vi "User ManualV1.vi"() -> ()   [LabVIEW 2020, in "Exaprom PDF.lvlib"]
uses:
  <userlib>/labview-PDF-writer-master/Exaprom PDF.lvlib
  <userlib>/labview-PDF-writer-master/Controls/Initialization Controls/Captions.ctl
  <userlib>/labview-PDF-writer-master/Controls/Initialization Controls/Image or Table Caption.ctl
  <userlib>/labview-PDF-writer-master/Controls/Font Controls/Font complete cluster.ctl
  <userlib>/labview-PDF-writer-master/Controls/Font Controls/Font size.ctl
  <userlib>/labview-PDF-writer-master/Controls/Font Controls/Font color.ctl
  <userlib>/labview-PDF-writer-master/Controls/Font Controls/Type and encoding.ctl
  <userlib>/labview-PDF-writer-master/Controls/Text Controls/Unicode/Type and run direction.ctl
  <userlib>/labview-PDF-writer-master/Controls/Initialization Controls/At the opening.ctl
  <userlib>/labview-PDF-writer-master/Controls/Initialization Controls/Defaut Paragraphe and Line Spacing.ctl
  <userlib>/labview-PDF-writer-master/Controls/Text Controls/Texte alignement.ctl
  <userlib>/labview-PDF-writer-master/Controls/Text Controls/Line spacing.ctl
  <userlib>/labview-PDF-writer-master/Controls/Initialization Controls/Unit.ctl
  <userlib>/labview-PDF-writer-master/Controls/Page Controls/Page setup.ctl
  <userlib>/labview-PDF-writer-master/Controls/Page Controls/Page size.ctl
  <userlib>/labview-PDF-writer-master/Controls/Page Controls/Page Orientation.ctl
  <userlib>/labview-PDF-writer-master/Controls/Page Controls/Page Layout Custom.ctl
  <userlib>/labview-PDF-writer-master/Controls/Page Controls/Page margins.ctl
  <userlib>/labview-PDF-writer-master/Controls/Image Controls/Image border.ctl
  <userlib>/labview-PDF-writer-master/Controls/Image Controls/Image alignment and position.ctl
  <userlib>/labview-PDF-writer-master/Controls/Image Controls/Image aligment.ctl
  <vilib>/measure/NI_MABase.lvlib
panel:
  out "波形图表":waveform(dbl)(graph)
  in  "Captions":T1={"Figure"={"Caption"="Figure", "Separator"=" QWE ", "Position"=enum."Below"}, "Table"={"Caption"="Table", "Separator"="  ", "Position"=enum."Above"}, "Font"={"Name"="", "Size"=-1.0, "Color"=0, "Style"={"Bold"=FALSE, "Italic"=FALSE, "Underline"=FALSE, "Strikeout"=FALSE}, "Type"={"Type&direction"=enum."Select", "Embedded"=FALSE, "Encoding"=""}}} caption="标题"
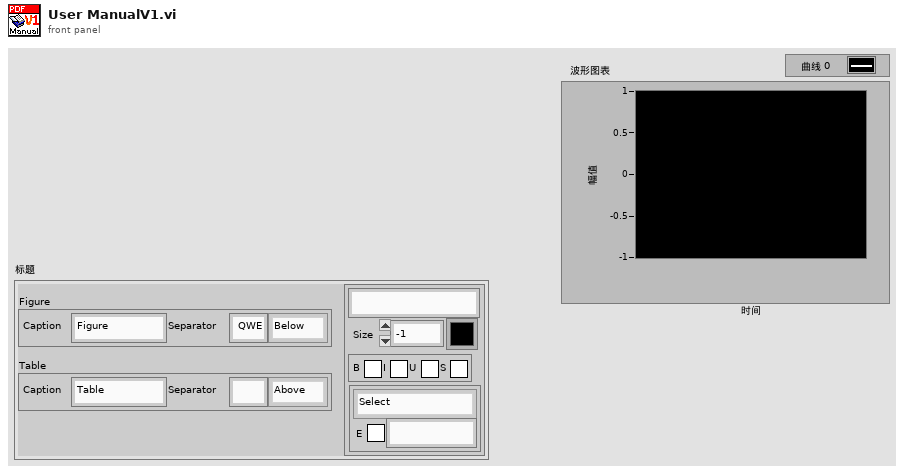
[diagram p1: front panel]
types:
  T1 = typedef "Exaprom PDF.lvlib/Captions.ctl" = cluster{"Figure":T2, "Table":T2, "Font":T3}
  T2 = typedef "Exaprom PDF.lvlib/Image or Table Caption.ctl" = cluster{"Caption":string, "Separator":string, "Position":enum16{"Above", "Below"}}
  T3 = typedef "Exaprom PDF.lvlib/Font complete cluster.ctl" = cluster{"Name":string, "Size":T4, "Color":T5, "Style":cluster{"Bold":bool, "Italic":bool, "Underline":bool, "Strikeout":bool}, "Type":T6}
  T4 = typedef "Exaprom PDF.lvlib/Font size.ctl" = sgl
  T5 = typedef "Exaprom PDF.lvlib/Font color.ctl" = u32
  T6 = typedef "Exaprom PDF.lvlib/Type and encoding.ctl" = cluster{"Type&direction":T7, "Embedded":bool, "Encoding":string}
  T7 = typedef "Exaprom PDF.lvlib/Type and run direction.ctl" = enum16{"Select", "ASCII", "UTF-16", "UTF-16 (default)", "UTF-16 (LTR)", "UTF-16 (RTL)"}
  T8 = typedef "Exaprom PDF.lvlib/Image alignment and position.ctl" = cluster{"Alignment":T9, "X ":sgl, "Y":sgl, "Indentation":sgl}
  T9 = typedef "Exaprom PDF.lvlib/Image aligment.ctl" = enum16{"Absolute (X,Y)", "Left", "Center", "Right", "Left (textwrap)", "Right (textwrap)"}
  T10 = typedef "Exaprom PDF.lvlib/Image border.ctl" = cluster{"Show?":bool, "Thickness (point)":sgl, "Color":u32}
  T11 = typedef "Exaprom PDF.lvlib/Page setup.ctl" = cluster{"Page Size":T12, "Orientation":T13, "Custom Size":T14, "Margins":T15}
  T12 = typedef "Exaprom PDF.lvlib/Page size.ctl" = i32
  T13 = typedef "Exaprom PDF.lvlib/Page Orientation.ctl" = enum16{"Portrait", "Landscape"}
  T14 = typedef "Exaprom PDF.lvlib/Page Layout Custom.ctl" = cluster{"Width":sgl, "Height":sgl}
  T15 = typedef "Exaprom PDF.lvlib/Page margins.ctl" = cluster{"Left":sgl, "Right":sgl, "Top":sgl, "Bottom":sgl}
  T16 = typedef "Exaprom PDF.lvlib/Unit.ctl" = enum16{"inch", "mm"}
  T17 = typedef "Exaprom PDF.lvlib/Defaut Paragraphe and Line Spacing.ctl" = cluster{" Aligment":T18, "Line spacing":T19}
  T18 = typedef "Exaprom PDF.lvlib/Texte alignement.ctl" = enum16{"Select", "CENTER", "JUSTIFY", "LEFT", "RIGHT"}
  T19 = typedef "Exaprom PDF.lvlib/Line spacing.ctl" = enum16{"Select", "1.0", "1.5", "2.0"}
  T20 = typedef "Exaprom PDF.lvlib/At the opening.ctl" = cluster{"Page":u16, "Show Bookmarks":bool}
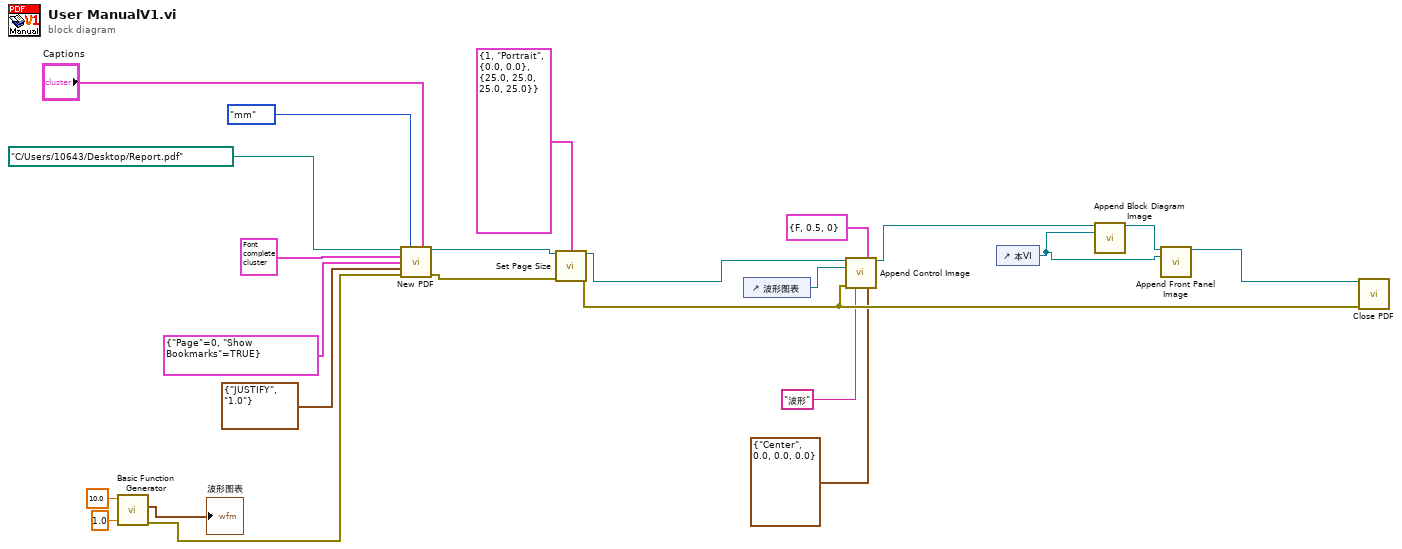
[diagram p0: block diagram]
diagram:
  n1 = call <vilib>:"Basic Function Generator.vi"("amplitude"=1.0, "frequency"=10.0) -> ("error out"=w8:errorcluster, "signal out"=→"波形图表":waveform(dbl))  [unwired: 7 in, 1 out]
  n2 = call <userlib>:"New PDF.vi"("PDF Path"=path "C:/Users/10643/Desktop/Report.pdf", "Unit (default = mm)"=Unit."mm", "Captions"="Captions", "Default Font"=T3 {"Name"="Arial", "Size"=12.0, "Color"=0, "Style"={"Bold"=FALSE, "Italic"=FALSE, "Underline"=FALSE, "Strikeout"=FALSE}, "Type"={"Type&direction"=enum."ASCII", "Embedded"=FALSE, "Encoding"=""}}, "At the opening"=T20 {"Page"=0, "Show Bookmarks"=TRUE}, "Default Paragraph"=T17 {" Aligment"=enum."JUSTIFY", "Line spacing"=enum."1.0"}, "error in (no error)"=w8) -> ("PDF Report"=w17:refnum<class "PDF Report Class.lvclass">, "error out"=w16:errorcluster)  [unwired: 7 in]
  n3 = call <userlib>:"Set Page Size.vi"("PDF Report IN"=w17, "Page setup"=T11 {"Page Size"=1, "Orientation"=enum."Portrait", "Custom Size"={"Width"=0.0, "Height"=0.0}, "Margins"={"Left"=25.0, "Right"=25.0, "Top"=25.0, "Bottom"=25.0}}, "error in (no error)"=w16) -> ("PDF Report OUT"=w14:refnum<class "PDF Report Class.lvclass">, "error OUT"=w13:errorcluster)  [unwired: 11 in]
  n4 = control-ref of="波形图表"() -> (w12:refnum<vi>)
  n5 = call <userlib>:"Append Control Image.vi"("PDF Report IN"=w14, "Border"=T10 {"Show?"=FALSE, "Thickness (point)"=0.5, "Color"=0}, "Ctrl reference"=w12, "error in (no error)"=w13, "Caption"="波形", "Position and indentation"=T8 {"Alignment"=enum."Center", "X "=0.0, "Y"=0.0, "Indentation"=0.0}) -> ("PDF Report OUT"=w4:refnum<class "PDF Report Class.lvclass">)  [unwired: 8 in, 1 out]
  n6 = control-ref of="本VI"() -> (w1:refnum<vi>)
  n7 = call <userlib>:"Append Block Diagram Image.vi"("PDF Report IN"=w4, "VI reference"=w1) -> ("PDF Report OUT"=w3:refnum<class "PDF Report Class.lvclass">)  [unwired: 12 in, 1 out]
  n8 = call <userlib>:"Append Front Panel Image.vi"("PDF Report IN"=w3, "VI reference"=w1) -> ("PDF Report OUT"=w2:refnum<class "PDF Report Class.lvclass">)  [unwired: 12 in, 1 out]
  n9 = call <userlib>:"Close PDF.vi"("PDF Report"=w2, "error in (no error)"=w13) -> ()  [unwired: 12 in, 2 out]
